vi "Read INI Cluster.vi"(8 "error in (no error)":errorcluster, 10 "INI Fomatted Cluster Type":variant, 11 "refnum":T1) -> (0 "error out":errorcluster, 1 "all found?":bool, 2 "INI Fomatted Cluster":variant, 3 "dup refnum":T1, 4 "any found?":bool)   [LabVIEW 2017, in "OpenG Variant Configuration File.lvlib"]
doc: "Reads a cluster of section formatted clusters from configuration data identified by refnum, and returns them as a cluster of clusters of items. Section cluster names are used as section names and key-value pairs correspond to the named cluster elements and thier values within the section formatted clusters. Only the section clusters and items within the \"INI Formatted Cluster Type\" input cluster are read from the configuration data and returned in the output cluster of clusters of items. The \"found?\" output will be TRUE only if all elements (recursively) are found.\n\nFor example an Cluster containins subClusters MyCluster1 and MyCluster2, where MyCluster1 contains two elements MyNumeric and MyBoolean, and MyCluster2 contains two elements MyEnum and MyString. This would correspond to an INI write of the following data:\n\n[MyCluster1]\nMyNumeric=1.024\nMyBoolean=TRUE\n[MyCluster2]\nMyEnum=init\nMyString=\"Hello World\"\n\nNote: Special characters in section and key names will be escape-coded. These include the following: \\00-\\1F (non-printable chars); \"[\", \"]\", and \"=\" (INI syntax elements); \\FE (\"þ\") and \\FF (\"ÿ\") (legacy bracket encoding); Additionally, the escape character, \"\\\", will be escaped as \"\\\\\".\n\nNote: This VI checks whether every element of the cluster has a name so it can be identified."
uses:
  OpenG Variant Configuration File.lvlib
  <vilib>/Utility/config.llb/Config Data RefNum.ctl
  _openG/_reuse_openG.lvlib
  <vilib>/Utility/Data Type/NI_Data Type.lvlib
  <vilib>/Utility/config.llb/NI_LVConfig.lvlib
panel:
  # "Read INI Cluster.vi\n\nReads a cluster (variant) of INI section clusters from INI file.\n\nPlease visit http://www.OpenG.org to learn about the\nOpen Source LabVIEW software movement.\n\nNOTICE -- YOU MUST LEAVE THIS NOTICE IN PLACE.  PER THE TERMS OF THE LICENSE BELOW, YOU MAY SUBLICENSE THIS SOFTWARE \nIN ANY WAY THAT DOES NOT CONFLICT WITH THIS LICENSE.\n\n### BSD License (http://www.opensource.org/licenses/bsd-license.php) Begin ###\n \nCopyright (c) 2002-2006, Jim Kring <jim@jimkring.com>\n\nAll rights reserved.\n\nRedistribution and use in source and binary forms, with or without modification, are permitted provided that the following conditions are met:\n\n    * Redistributions of source code must retain the above copyright notice, this list of conditions and the following disclaimer.\n    * Redistributions in binary form must reproduce the above copyright notice, this list of conditions and the following disclaimer in the \n       documentation and/or other materials provided with the distribution.\n    * Neither the name of SciWare, James Kring, Inc., nor the names of its contributors may be used to endorse or promote products derived \n       from this software without specific prior written permission.\n\nTHIS SOFTWARE IS PROVIDED BY THE COPYRIGHT HOLDERS AND CONTRIBUTORS \"AS IS\" AND ANY EXPRESS OR IMPLIED WARRANTIES, \nINCLUDING, BUT NOT LIMITED TO, THE IMPLIED WARRANTIES OF MERCHANTABILITY AND FITNESS FOR A PARTICULAR PURPOSE ARE \nDISCLAIMED. IN NO EVENT SHALL THE COPYRIGHT OWNER OR CONTRIBUTORS BE LIABLE FOR ANY DIRECT, INDIRECT, INCIDENTAL,\n SPECIAL, EXEMPLARY, OR CONSEQUENTIAL DAMAGES (INCLUDING, BUT NOT LIMITED TO, PROCUREMENT OF SUBSTITUTE GOODS OR \nSERVICES; LOSS OF USE, DATA, OR PROFITS; OR BUSINESS INTERRUPTION) HOWEVER CAUSED AND ON ANY THEORY OF LIABILITY, \nWHETHER IN CONTRACT, STRICT LIABILITY, OR TORT (INCLUDING NEGLIGENCE OR OTHERWISE) ARISING IN ANY WAY OUT OF THE USE \nOF THIS SOFTWARE, EVEN IF ADVISED OF THE POSSIBILITY OF SUCH DAMAGE.\n\n### BSD License End ###"
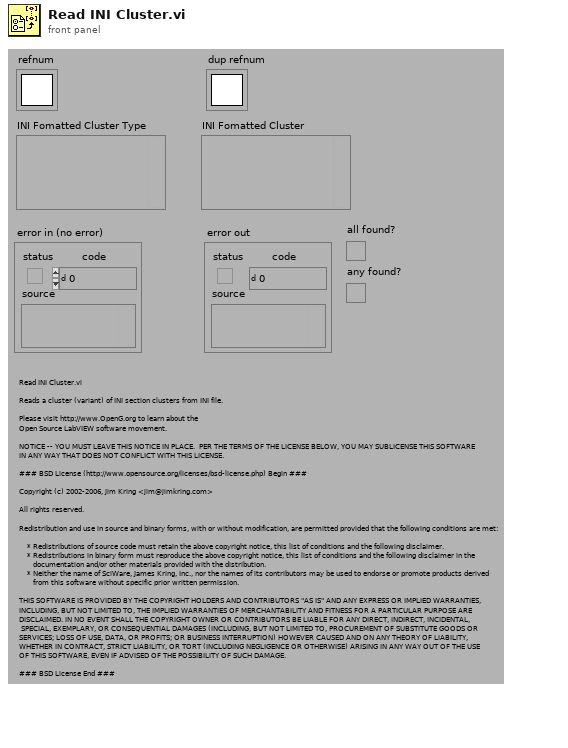
[diagram p1: front panel]
types:
  T1 = typedef "NI_LVConfig.lvlib/Config Data RefNum.ctl" = refnum<k1>
  T2 = typedef "NI_Data Type.lvlib/Data Type.ctl" = enum8{"Invalid Type", "Void", "I8", "I16", "I32", "I64", "U8", "U16", "U32", "U64", "Single Float", "Double Float", "Extended Float", "Single Complex", "Double Complex", "Extended Complex", "Enum U8", "Enum U16", "Enum U32", "Enum U64", "Single Float With Unit", "Double Float With Unit", "Extended Float With Unit", "Single Complex with Unit", "Double Complex with Unit", "Extended Complex with Unit", "Boolean", "String", "Path", "Picture", "Tag", "Array", "Cluster", "Variant", "LV Variant", "Waveform", "Timestamp", "Digital Waveform", "Digital Data", "ExpressData", "Refnum", "External Data", "VI", "Poly VI", "LabVIEW Class Instance", "Fixed Point"}
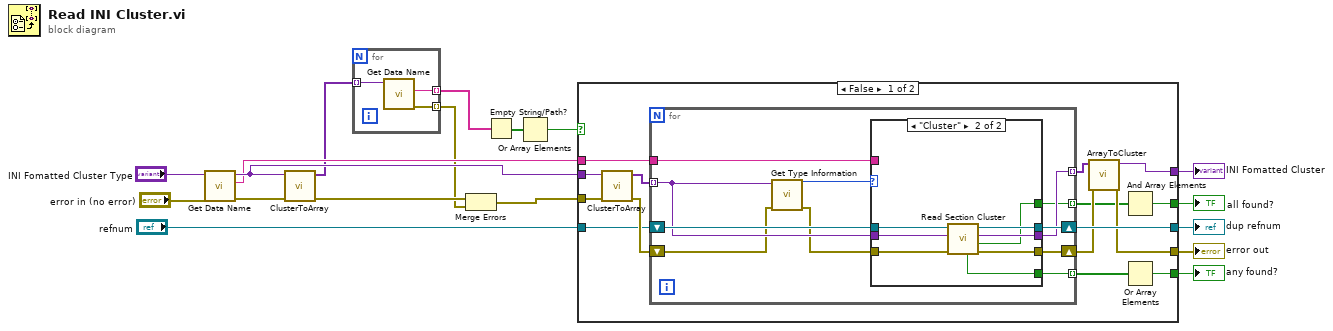
[diagram p0: block diagram]
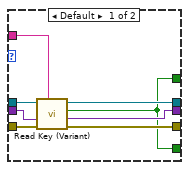
[diagram p2: hidden frame]
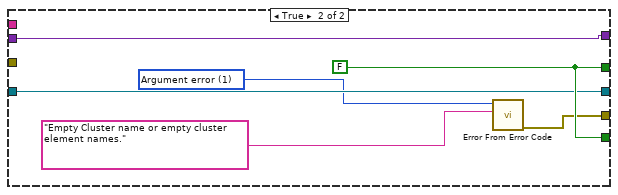
[diagram p3: hidden frame]
diagram:
  n1 = call "Get Data Name.vi"("error in (no error)"="error in (no error)", "Data"="INI Fomatted Cluster Type") -> ("error out"=w8:errorcluster, "Data Name"=w7:string, "Data Dup"=w9:variant)  [unwired: 7 in]
  n2 = call "ClusterToArray.vi"("Error in"=w8, "Cluster"=w9) -> ("Error out"=w5:errorcluster, "Array"=w4:variant[])  [unwired: 8 in]
  n3 = for {
    tunnel: w4 -> [w21] mode=indexing
    tunnel: [w20] -> w3 mode=indexing
    tunnel: [w19] -> w1 mode=indexing
    n4 = call "Get Data Name.vi"("Data"=w21) -> ("error out"=w19:errorcluster, "Data Name"=w20:string)  [unwired: 8 in, 1 out]
  }
  n5 = Merge Errors(w5, w1) -> (w2:errorcluster)
  n6 = Empty String/Path?(string/path=w3) -> (empty?=w10:bool[])
  n7 = Or Array Elements(Boolean array=w10) -> (logical OR=w6:bool)
  n8 = case shown="False" w6 {
    tunnel: [w35 w67] -> w18
    tunnel: "refnum" -> [w34 w67]
    tunnel: [w31 w69] -> w16
    tunnel: [w29 w64] -> w13
    tunnel: [w28 w68] -> w12
    tunnel: [w27 w68] -> w11
    tunnel: w9 -> [w24 w69]
    tunnel: w7 -> [w23 _]
    tunnel: w2 -> [w22 _]
    frame False {
      n9 = call "ClusterToArray.vi"("Error in"=w22, "Cluster"=w24) -> ("Error out"=w36:errorcluster, "Array"=w33:variant[])  [unwired: 8 in]
      n10 = for {
        tunnel: w33 -> [w43] mode=indexing
        shift-right: [w45] -> w35
        shift-left: w34 -> [w47]
        shift-right: [w46] -> w30
        shift-left: w36 -> [w38]
        tunnel: [w44] -> w32 mode=indexing
        tunnel: w23 -> [w41]
        tunnel: [w40] -> w25 mode=indexing
        tunnel: [w39] -> w26 mode=indexing
        n11 = call <vilib>:"Get Type Information.vi"("error in (no error)"=w38, "Variant"=w43) -> ("error out"=w37:errorcluster, "Type"=w42:T2)  [unwired: 5 in, 3 out]
        n12 = case shown="\"Cluster\"" w42 {
          tunnel: w47 -> [w53 w63]
          tunnel: w37 -> [w55 w62]
          tunnel: [w54 w61] -> w46
          tunnel: [w50 w60] -> w45
          tunnel: [w51 w59] -> w44
          tunnel: w43 -> [w49 w58]
          tunnel: w41 -> [w52 _]
          tunnel: [w48 w57] -> w40
          tunnel: [w48 w56] -> w39
          frame Default {
            n13 = call "Read Key (Variant).vi"("section"=w52, "error in (no error)"=w55, "type"=w49, "refnum"=w53) -> ("error out"=w54:errorcluster, "key-value"=w51:variant, "found?"=w48:bool, "refnum out"=w50:T1)  [unwired: 4 in]
          }
          frame "Cluster" {
            n14 = call "Read Section Cluster.vi"("error in (no error)"=w62, "Section Formatted Cluster Type"=w58, "refnum"=w63) -> ("error out"=w61:errorcluster, "all found?"=w57:bool, "Section Formatted Cluster"=w59:variant, "dup refnum"=w60:T1, "any found?"=w56:bool)  [unwired: 4 in]
          }
        }
      }
      n15 = call "ArrayToCluster.vi"("Error in"=w30, "Array"=w32) -> ("Error out"=w29:errorcluster, "Cluster"=w31:variant)  [unwired: 8 in]
      n16 = And Array Elements(Boolean array=w25) -> (logical AND=w28:bool)
      n17 = Or Array Elements(Boolean array=w26) -> (logical OR=w27:bool)
    }
    frame True {
      w66 = 1 items=["No error", "Argument error", "Memory is full", "Out of zone", "End of file", "File already open", "Generic file I/O error", "File not found", "File permission error", "Disk is full", "Duplicate path", "Too many files open", "System feature not enabled", "Resource file not found", "Cannot add resource", "Resource not found", "Image not found", "Image memory error", "Pen does not exist", "Config type invalid", "Config token not found", "Config parse error", "Config memory error", "Bad external code format", "Bad external code offset", "External code not present", "Null window", "Destroy window error", "Null menu", "Print aborted", "Bad print record", "Print driver error", "Windows error during printing", "Memory error during printing", "Print dialog error", "Generic print error", "Invalid device refnum", "Device not found", "Device parameter error", "Device unit error", "Cannot open device", "Device call aborted", "Generic error", "Cancelled by user", "Object ID too low", "Object ID too high", "Object not in heap", "Unknown heap", "Unknown object (invalid DefProc)", "Unknown object (DefProc not in table)", "Message out of range", "Invalid (null) method", "Unknown message", "Manager call not supported", "Bad address", "Network operation in progress", "Network operation timed out", "Connection is busy", "Network attribute not supported", "Network error", "Address in use", "System out of memory", "Connection aborted", "Connection refused", "Not connected", "Already connected", "Connection closed", "Initialization error (interapplication manager)", "Bad occurrence", "Wait on unbound occurrence handler", "Occurrence queue overflow", "Datalog type conflict", "Unused", "Unrecognized type (interapplication manager)", "Memory corrupt", "Failed to make temporary DLL", "Old CIN version", "Drag socket not found", "Failed to load drop-object", "Failed to register OLE object", "Failed to release OLE object", "Format specifier type mismatch", "Unknown format specifier", "Too few format specifiers", "Too many format specifiers", "Scan failed", "Newer CIN version", "Error converting to variant", "Runtime menu error", "Password tampered", "Variant attribute not found", "Incompatible variant data type", "Event data is not available", "Event Store is not present", "Occurrence is not found", "Event Queue is not created", "Event info is not available", "Refnum passed is NULL", "Error retrieving Class GUID", "Error retrieving CoClass GUID", "Error retrieving TypeLib GUID.", "Bad built application magic bytes.", "Specific driver is different from the specific driver associated with the Logical Name.", "There is no session opened to the class driver.", "Max Error", "MAX - Error with config objects", "MAX - Error loading configuration", "MAX - Group not supported"]
      w68 = FALSE
      n18 = call "Error From Error Code.vi"("error message (\"\")"="Empty Cluster name or empty cluster element names." ("String to Prepend to source (\"\")"), "error code (0)"=w66) -> ("error out"=w64:errorcluster)  [unwired: 7 in]
    }
  }
  "error out" <- w13
  "dup refnum" <- w18
  "INI Fomatted Cluster" <- w16
  "all found?" <- w12
  "any found?" <- w11
